vi "Module Running as Cloneable--error.vi"() -> (0 "error out":errorcluster)   [LabVIEW 2020, in "Client HTTP Get.lvlib"]
doc: "Outputs an error cluster containing a custom error code indicating the module was running as a cloneable, but Start Module has the 'Run as Singleton' input set to TRUE.\n_____\nBased on DQMH Project Template 6.0.0.91."
uses:
  Client HTTP Get.lvlib
  <vilib>/Utility/error.llb/Error Cluster From Error Code.vi
  <vilib>/ErrorRing/Error Ring.xnode
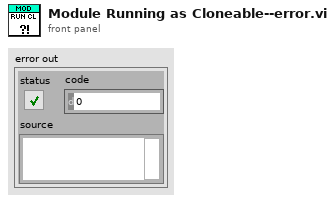
[diagram p1: front panel]
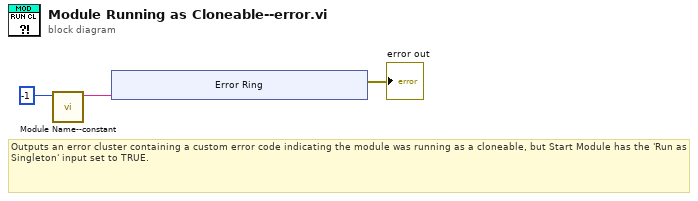
[diagram p0: block diagram]
diagram:
  # "Outputs an error cluster containing a custom error code indicating the module was running as a cloneable, but Start Module has the 'Run as Singleton' input set to TRUE."
  n1 = call "Module Name--constant.vi"("Module ID"=-1) -> ("Module Name"=w2:string)  [unwired: 10 in]
  n2 = xnode "Error Ring"("parameter 0"=w2) -> ("error out"=→"error out":errorcluster)
